vi "Microscope.InitializeInstrument.vi"(8 "error in (no error)":errorcluster, 9 "timeout (5000 ms)":i32=5000, 11 "Microscope":refnum<class "Microscope.lvclass">) -> (0 "error out":errorcluster, 1 "Init complete":bool, 3 "Microscope out":refnum<class "Microscope.lvclass">)   [LabVIEW 2013, in "Microscope.lvclass"]
doc: "---------------------------------------------------------------\nJKI State Machine Objects™\nhttp://jki.net/state-machine-objects/\nCopyright (C) 2005-2015, JKI <info@jki.net>\nALL RIGHTS RESERVEDJKI State Machine Objects (SMO) 1.0.0.5\nJKI - JKI\nCopyright (c) 2016, JKI"
uses:
  Microscope.lvclass
  XYStage/XYStage.lvclass
panel:
  # "For instructions on how to use the JKI State Machine Objects, examples and video tutorials, visit:\nhttp://jki.net/state-machine-objects/\n\nJKI State Machine Objects™\nhttp://jki.net/state-machine-objects/\nCopyright (C) 2005-2015, JKI <info@jki.net>\nALL RIGHTS RESERVED"
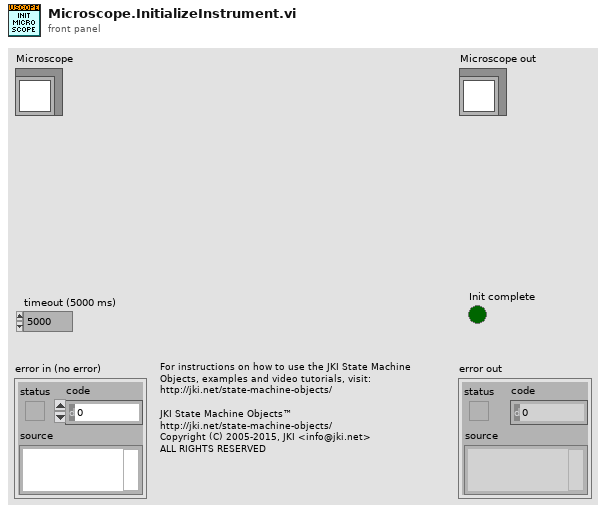
[diagram p1: front panel]
types:
  T1 = typedef "Microscope.lvclass/Dependencies--Cluster.ctl" = cluster{"XYStage":refnum<class "XYStage.lvclass">, "Camera":refnum<class "Camera.lvclass">}
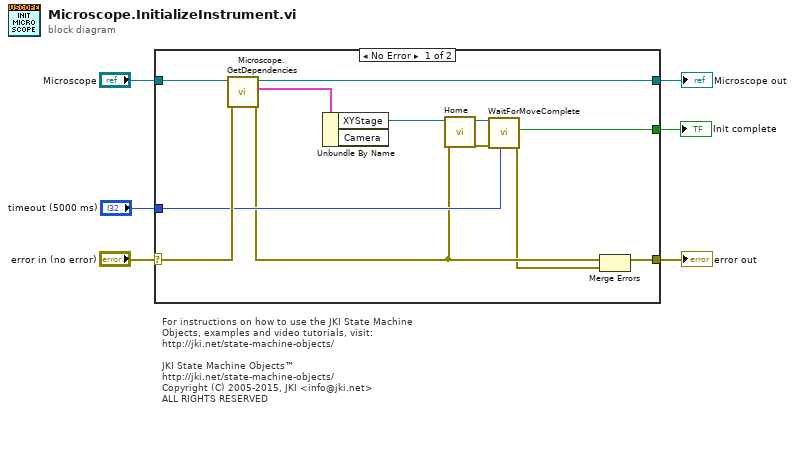
[diagram p0: block diagram]
diagram:
  # "For instructions on how to use the JKI State Machine Objects, examples and video tutorials, visit:\nhttp://jki.net/state-machine-objects/\n\nJKI State Machine Objects™\nhttp://jki.net/state-machine-objects/\nCopyright (C) 2005-2015, JKI <info@jki.net>\nALL RIGHTS RESERVED"
  n1 = case shown="No Error" "error in (no error)" {
    selector: "error in (no error)" -> [w17 w19]
    tunnel: "Microscope" -> [w18 w20]
    tunnel: [w7 w19] -> w5
    tunnel: [w16 w20] -> w4
    tunnel: [w12 _] -> w1
    tunnel: "timeout (5000 ms)" -> [w11 _]
    frame No Error {
      n2 = call "Microscope.GetDependencies.vi"("error in (no error)"=w17, "Microscope"=w18) -> ("error out"=w10:errorcluster, "Dependencies"=w15:T1, "Microscope out"=w16:refnum<class "Microscope.lvclass">)  [unwired: 7 in]
      n3 = Unbundle By Name(w15) -> ("XYStage"=w14:refnum<class "XYStage.lvclass">)  [unwired: 1 out]
      n4 = call "Home.vi"("error in (no error)"=w10, "XYStage"=w14) -> ("error out"=w9:errorcluster, "XYStage out"=w13:refnum<class "XYStage.lvclass">)  [unwired: 8 in]
      n5 = call "WaitForMoveComplete.vi"("timeout (5000 ms)"=w11, "error in (no error)"=w9, "XYStage"=w13) -> ("error out"=w8:errorcluster, "move complete"=w12:bool)  [unwired: 6 in, 1 out]
      n6 = Merge Errors(w10, w8) -> (w7:errorcluster)
    }
    frame Error {
    }
  }
  "error out" <- w5
  "Microscope out" <- w4
  "Init complete" <- w1
